vi "Test dispersion compensation.vi"() -> ()   [LabVIEW 2018]
uses:
  Hardware Mfg/AlazarTech SDK/Controls/Alazar Engine Actions.ctl
panel:
  out "Metric":dbl[](graph)
  out "indexsWhereTrue":i32[](array[numeric])
  in  "lessThan":i32=13
  out "x < y?":bool[](array[boolean])
  out "error out":errorcluster
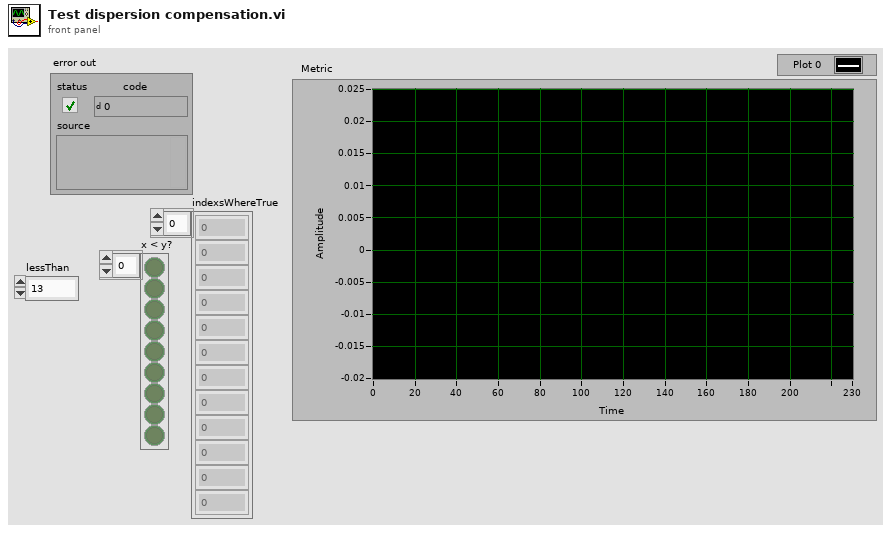
[diagram p1: front panel]
types:
  T1 = typedef "Alazar Engine Actions.ctl" = enum16{"Init", "Config Clock", "Config Ch", "Config Trig", "Config Non-FFT Acq.", "Non-FFT Acquire", "Load background from Non-FFT buffer", "enable background subtrac", "disable background subtrac", "load background from file", "load background from elsewhere", "start acquire", "background subtraction", "Config Acq.", "Acquire", "UnInit"}
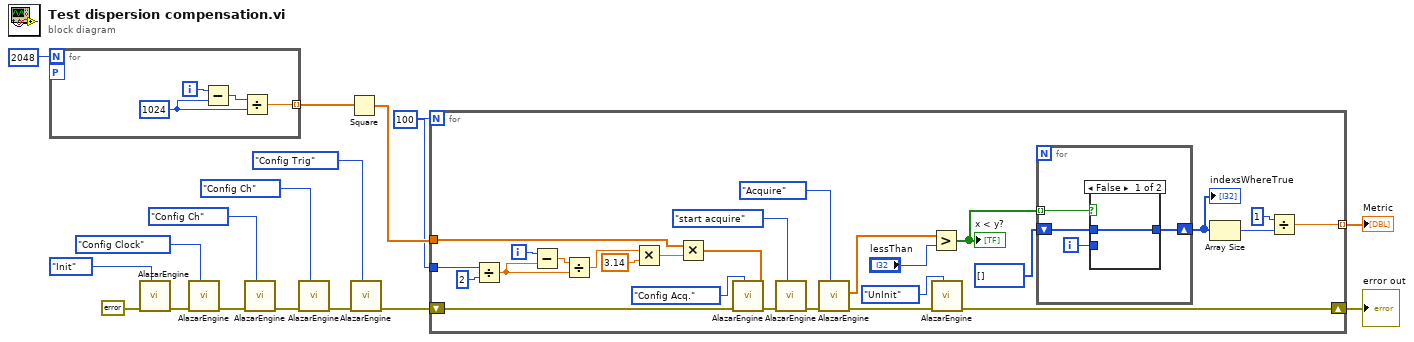
[diagram p0: block diagram]
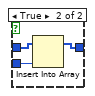
[diagram p2: hidden frame]
diagram:
  w2 = 100
  n1 = for {
    N: 2048 -> [_]
    tunnel: [w18] -> w4 mode=indexing
    workers-P: _ -> [_]
    i -> [w21]
    w19 = 1024 ("y")
    n2 = Subtract(x=w21, y=w19) -> (x-y=w20:i32)
    n3 = Divide(x=w20, y=w19) -> (x/y=w18:dbl)
  }
  n4 = call "AlazarEngine.vi"("Action"=Alazar_Engine_Actions."Init", "error in (no error)"=errorcluster {"status"=FALSE, "code"=0, "source"=""}) -> ("error out"=w16:errorcluster)  [unwired: 8 in, 1 out]
  n5 = call "AlazarEngine.vi"("Action"=Alazar_Engine_Actions."Config Clock", "error in (no error)"=w16) -> ("error out"=w15:errorcluster)  [unwired: 8 in, 1 out]
  n6 = call "AlazarEngine.vi"("Action"=Alazar_Engine_Actions."Config Ch", "error in (no error)"=w15) -> ("error out"=w14:errorcluster)  [unwired: 8 in, 1 out]
  n7 = call "AlazarEngine.vi"("Action"=Alazar_Engine_Actions."Config Ch", "error in (no error)"=w14) -> ("error out"=w13:errorcluster)  [unwired: 8 in, 1 out]
  n8 = Square(x=w4) -> (x^2=w3:dbl[])
  n9 = call "AlazarEngine.vi"("Action"=Alazar_Engine_Actions."Config Trig", "error in (no error)"=w13) -> ("error out"=w7:errorcluster)  [unwired: 8 in, 1 out]
  n10 = for {
    N: w2 -> [_]
    shift-right: [w40] -> w6
    shift-left: w7 -> [w44]
    tunnel: w3 -> [w34]
    tunnel: w2 -> [w39]
    tunnel: [w25] -> w1 mode=indexing
    i -> [w37]
    n11 = Divide(x=w39, y=2) -> (x/y=w35:dbl)
    n12 = Subtract(x=w37, y=w35) -> (x-y=w36:dbl)
    n13 = Divide(x=w36, y=w35) -> (x/y=w23:dbl)
    n14 = Multiply(x=w23, y=3.14) -> (x*y=w24:dbl)
    n15 = Multiply(x=w34, y=w24) -> (x*y=w33:dbl[])
    n16 = call "AlazarEngine.vi"("Imag window array"=w33, "Action"=Alazar_Engine_Actions."Config Acq.", "error in (no error)"=w44) -> ("error out"=w43:errorcluster)  [unwired: 7 in, 1 out]
    n17 = call "AlazarEngine.vi"("Action"=Alazar_Engine_Actions."start acquire", "error in (no error)"=w43) -> ("error out"=w42:errorcluster)  [unwired: 8 in, 1 out]
    n18 = call "AlazarEngine.vi"("Action"=Alazar_Engine_Actions."Acquire", "error in (no error)"=w42) -> ("error out"=w41:errorcluster, "Buffer"=w31:sgl[])  [unwired: 8 in]
    n19 = Greater?(x=w31, y="lessThan") -> (0:w29:bool[])
    "x < y?" <- w29
    n20 = call "AlazarEngine.vi"("Action"=Alazar_Engine_Actions."UnInit", "error in (no error)"=w41) -> ("error out"=w40:errorcluster)  [unwired: 8 in, 1 out]
    n21 = for {
      tunnel: w29 -> [w52] mode=indexing
      shift-right: [w49] -> w28
      shift-left: i32[] [] -> [w50]
      i -> [w51]
      n22 = case shown="False" w52 {
        tunnel: w51 -> [_ w55]
        tunnel: w50 -> [w53 w56]
        tunnel: [w53 w54] -> w49
        frame False {
        }
        frame True {
          n23 = Insert Into Array(array=w56, new element=w55) -> (w54:i32[])  [unwired: 1 in]
        }
      }
    }
    "indexsWhereTrue" <- w28
    n24 = Array Size(array=w28) -> (size(s)=w27:i32)
    n25 = Divide(x=1, y=w27) -> (x/y=w25:dbl)
  }
  "error out" <- w6
  "Metric" <- w1
